vi "Read Occurrence Ref.vi"(8 "error in (no error)":errorcluster, 11 "Without Data in":refnum<class "Without Data.lvclass">) -> (0 "error out":errorcluster, 2 "Occurrence Ref":refnum<k4>, 3 "Without Data out":refnum<class "Without Data.lvclass">)   [LabVIEW 2020, in "Without Data.lvclass"]
doc: "This is the parent VI which is used to get the occurrence reference"
uses:
  Classes/Children/Intra-Application/Children/Without data/Without Data.lvclass
  Classes/Children/Intra-Application/Children/Without data/Without Data.lvclass/Without Data.ctl
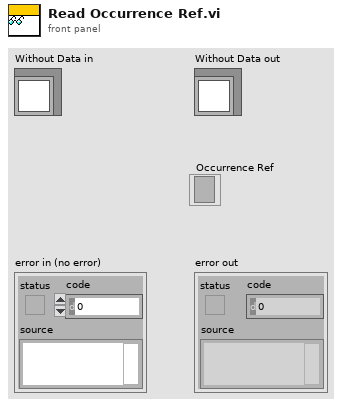
[diagram p1: front panel]
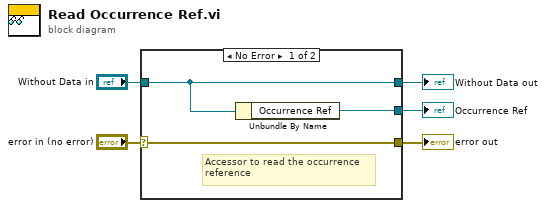
[diagram p0: block diagram]
diagram:
  n1 = case shown="No Error" "error in (no error)" {
    selector: "error in (no error)" -> [w8 w9]
    tunnel: [w8 w9] -> w4
    tunnel: [w7 w10] -> w2
    tunnel: "Without Data in" -> [w7 w10]
    tunnel: [w6 _] -> w1
    frame No Error {
      # "Accessor to read the occurrence\nreference"
      n2 = Unbundle By Name(w7) -> ("Occurrence Ref"=w6:refnum<k4>)
    }
    frame Error {
    }
  }
  "error out" <- w4
  "Without Data out" <- w2
  "Occurrence Ref" <- w1
